vi "Handle Error.vi"(8 "error in (no error)":errorcluster, 11 "Zero Timeout Message Handler in":refnum<class "Zero Timeout Message Handler.lvclass">) -> (0 "error out":errorcluster, 3 "Zero Timeout Message Handler out":refnum<class "Zero Timeout Message Handler.lvclass">, 4 "stop?":bool)   [LabVIEW 2024, in "Zero Timeout Message Handler.lvlib" / "Zero Timeout Message Handler.lvclass"]
uses:
  Zero Timeout Message Handler.lvclass
  Zero Timeout Message Handler.lvclass/Zero Timeout Message Handler.ctl
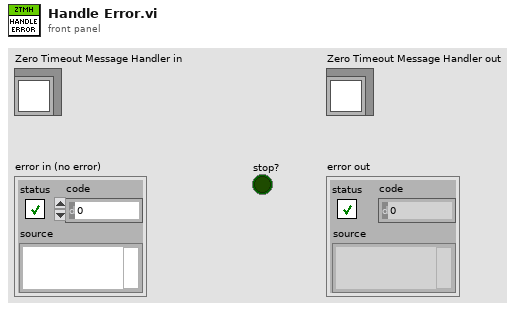
[diagram p1: front panel]
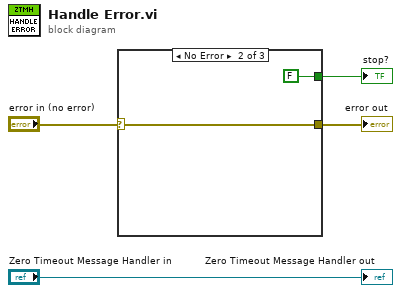
[diagram p0: block diagram]
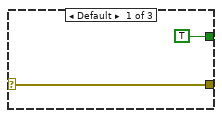
[diagram p2: hidden frame]
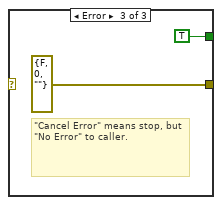
[diagram p3: hidden frame]
diagram:
  n1 = case shown="No Error" "error in (no error)" {
    selector: "error in (no error)" -> [w5 w7 _]
    tunnel: [w5 w7 errorcluster {"status"=FALSE, "code"=0, "source"=""} ("error IO")] -> w3
    tunnel: [TRUE FALSE TRUE] -> w1
    frame Default {
    }
    frame No Error {
    }
    frame Error {
      # "\"Cancel Error\" means stop, but \"No Error\" to caller."
    }
  }
  "error out" <- w3
  "stop?" <- w1
  "Zero Timeout Message Handler out" <- "Zero Timeout Message Handler in"
